vi "BinPicture4.vi"(1 "Binning size":i32=1, 2 "To bin":dbl[][](graph)=array172x130[22360 elements]) -> (0 "Output":dbl[][](graph))   [LabVIEW 2010]
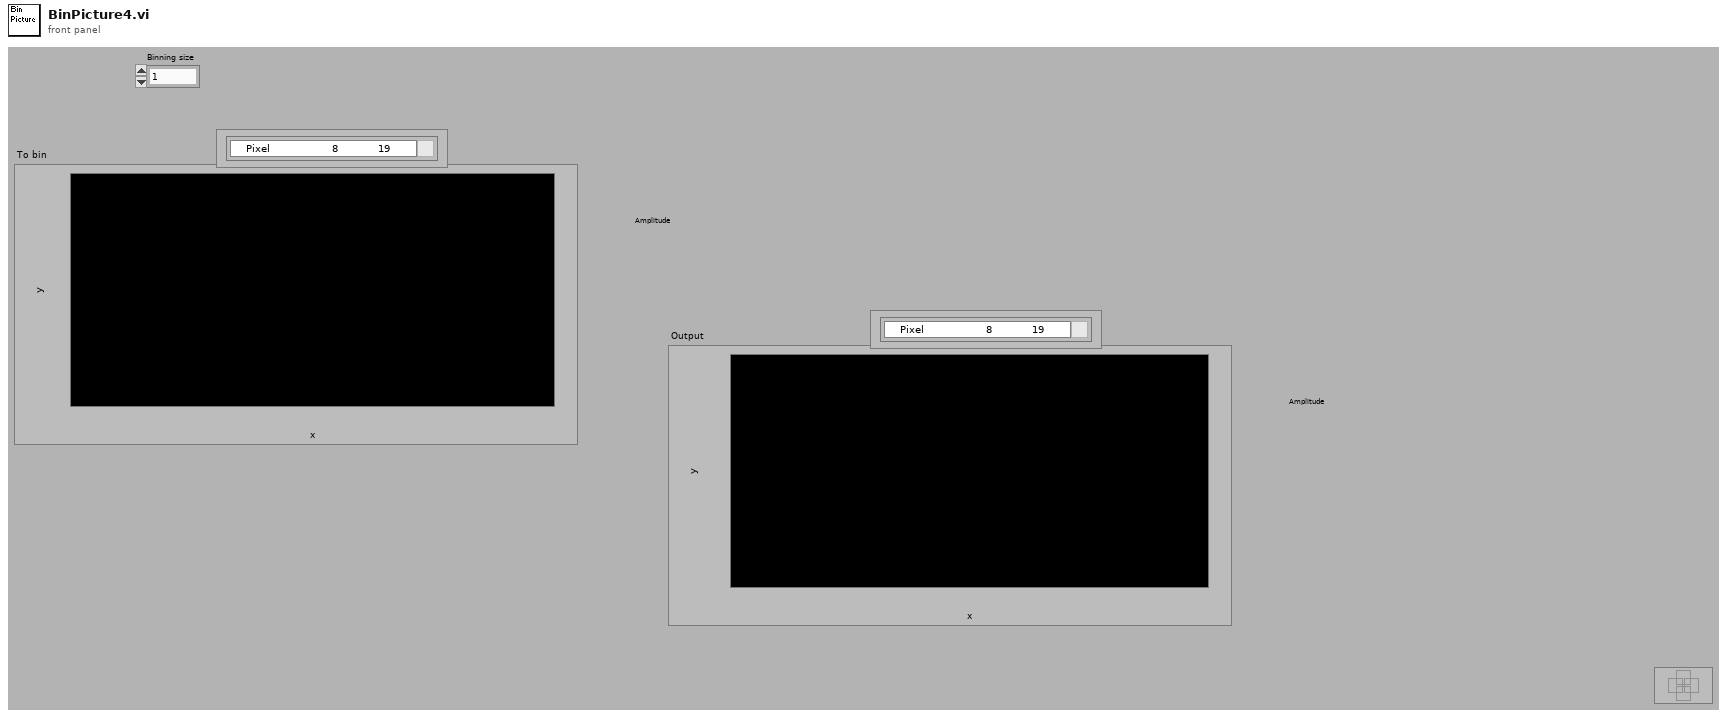
[diagram p1: front panel]
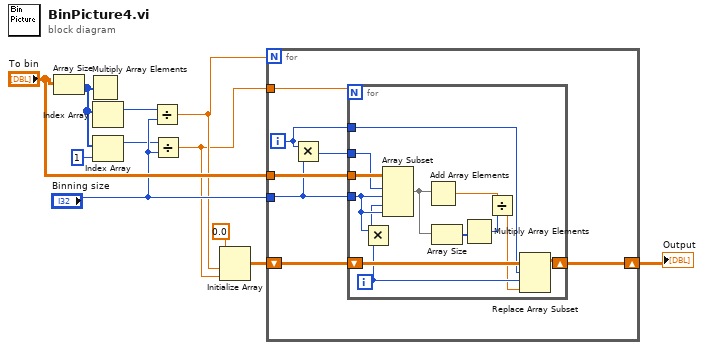
[diagram p0: block diagram]
diagram:
  n1 = Array Size(array="To bin") -> (size(s)=w10:i32[])
  n2 = Multiply Array Elements(1:w10) -> ()  [unwired: 1 out]
  n3 = Index Array(array=w10) -> (element=w6:i32)  [unwired: 1 in]
  n4 = Index Array(array=w10, index=1) -> (element=w7:i32)
  n5 = Divide(x=w6, y="Binning size") -> (x/y=w5:dbl)
  n6 = Divide(x=w7, y="Binning size") -> (x/y=w4:dbl)
  n7 = Initialize Array(0.0 ("element"), w5, w4) -> (w3:dbl[][])
  n8 = for {
    N: w5 -> [_]
    tunnel: "To bin" -> [w18]
    tunnel: "Binning size" -> [w16]
    tunnel: w4 -> [w17]
    shift-right: [w12] -> w1
    shift-left: w3 -> [w14]
    i -> [w13]
    n9 = Multiply(x=w13, y=w16) -> (x*y=w15:i32)
    n10 = for {
      N: w17 -> [_]
      tunnel: w18 -> [w31]
      tunnel: w16 -> [w30]
      tunnel: w15 -> [w28]
      tunnel: w13 -> [w21]
      shift-right: [w19] -> w12
      shift-left: w14 -> [w23]
      i -> [w22]
      n11 = Multiply(x=w30, y=w22) -> (x*y=w29:i32)
      n12 = Array Subset(array=w31, index (row)=w28, length (row)=w30, index (col)=w29, length (col)=w30) -> (w27:dbl[][])
      n13 = Add Array Elements(numeric array=w27) -> (sum=w24:dbl)
      n14 = Array Size(array=w27) -> (size(s)=w26:i32[])
      n15 = Multiply Array Elements(1:w26) -> (0:w25:i32)
      n16 = Divide(x=w24, y=w25) -> (x/y=w20:dbl)
      n17 = Replace Array Subset(array=w23, new element=w20, index (row)=w21, index (col)=w22) -> (w19:dbl[][])
    }
  }
  "Output" <- w1
